vi "MainAccelerometer.vi"() -> ()   [LabVIEW 2014]
uses:
  <vilib>/myRIO/Instrument Drivers/Onboard Devices/Accelerometer/typedefs/Accelerometer Reference.ctl
  <vilib>/myRIO/Common/Instrument Driver Framework/Utilities/typedefs/myRIO Generic Hardware Reference.ctl
  <vilib>/myRIO/Common/Instrument Driver Framework/Utilities/typedefs/Hardware Version Enum.ctl
  <vilib>/myRIO/Common/Instrument Driver Framework/Utilities/typedefs/myRIO v1.0 Reference.ctl
  <vilib>/myRIO/Common/Instrument Driver Framework/Utilities/typedefs/Generic FPGA Reference.ctl
  <vilib>/myRIO/Common/Instrument Driver Framework/myRIO v1.0/Accelerometer/typedefs/Accelerometer Channels List.ctl
  <vilib>/myRIO/Common/Instrument Driver Framework/myRIO v1.0/Accelerometer/typedefs/Accelerometer Channels Enum.ctl
  <vilib>/userdefined/High Color/nirio_resource_hc.ctl
  <vilib>/myRIO/Common/Instrument Driver Framework/Utilities/vis/Is FPGA Ref Available.vi
  <vilib>/myRIO/Common/Instrument Driver Framework/myRIO v1.0/Accelerometer/vis/myRIO v1.1 Open Accelerometer.vi
  <vilib>/myRIO/Instrument Drivers/Onboard Devices/Accelerometer/vis/Read.vi
  <vilib>/myRIO/Common/Instrument Driver Framework/Utilities/vis/Validate Channels.vi
  <vilib>/myRIO/Common/Instrument Driver Framework/myRIO v1.0/Accelerometer/vis/myRIO v1.0 Reserve Accelerometer.vi
  <vilib>/myRIO/Common/Instrument Driver Framework/myRIO v1.0/UART/vis/myRIO v1.0 Close UART.vi
  <vilib>/myRIO/Common/Instrument Driver Framework/myRIO v1.0/Resource Manager/vis/myRIO v1.0 Reserve Channel List.vi
  <vilib>/myRIO/Common/Instrument Driver Framework/myRIO v1.0/Accelerometer/vis/myRIO v1.0 Build MUX Configuration Accelerometer.vi
  <vilib>/myRIO/Common/Instrument Driver Framework/myRIO v1.0/Resource Manager/vis/myRIO v1.0 Reserve Channel.vi
  <vilib>/myRIO/Common/Instrument Driver Framework/myRIO v1.0/Resource Manager/vis/myRIO v1.0 Unreserve Channel.vi
  <vilib>/myRIO/Common/Instrument Driver Framework/myRIO v1.0/Resource Manager/vis/myRIO v1.0 Build Mutex Name.vi
  <vilib>/Utility/VariantDataType/GetNumericInfo.vi
  <vilib>/Utility/error.llb/Error Cluster From Error Code.vi
  <vilib>/myRIO/Common/Instrument Driver Framework/myRIO v1.0/myRIO v1.1 Open.vi
  <vilib>/myRIO/Common/Instrument Driver Framework/myRIO v1.0/Accelerometer/vis/myRIO v1.0 Get Scaling Constant Accelerometer.vi
  <vilib>/myRIO/Common/Instrument Driver Framework/Utilities/vis/IO Manager.vi
  <vilib>/myRIO/Common/Instrument Driver Framework/Utilities/vis/Configuration Manager.vi
  <vilib>/myRIO/Common/Instrument Driver Framework/myRIO v1.0/myRIO v1.0 Close.vi
  <vilib>/myRIO/Common/Instrument Driver Framework/myRIO v1.0/Accelerometer/vis/myRIO v1.0 Read Accelerometer.vi
  <vilib>/myRIO/Common/Instrument Driver Framework/Utilities/vis/FPGA Ref Manager.vi
  <vilib>/myRIO/Common/Instrument Driver Framework/myRIO v1.0/myRIO v1.0 Reset FPGA.vi
  <vilib>/myRIO/Common/Instrument Driver Framework/myRIO v1.0/IRQ/vis/myRIO v1.0 IRQ Info FGV.vi
  <vilib>/myRIO/Common/Instrument Driver Framework/myRIO v1.0/IRQ/vis/myRIO v1.0 Timer IRQ Info FGV.vi
  <vilib>/myRIO/Common/Instrument Driver Framework/myRIO v1.0/IRQ/vis/myRIO v1.0 ISR Agent.vi
  <vilib>/myRIO/Express VI/Onboard Devices/Accelerometer/Accelerometer Express VI.xnode
  <vilib>/myRIO/Instrument Drivers/Onboard Devices/Accelerometer/vis/myRIO Accelerometer Open.xnode
  <vilib>/myRIO/Instrument Drivers/Utilities/Utilities.lvlib
  <vilib>/myRIO/Instrument Drivers/Onboard Devices/Accelerometer/Accelerometer.lvlib
panel:
  out "Acceleration":T1(graph)
  out "error out":errorcluster
  in  "Stop Button":bool
  # "Overview: The myRIO Project template acquires acceleration data from the onboard accelerometer and displays the changes of acceleration values in a waveform chart.\nInstructions:\n1. Check the myRIO target IP Address in the project and make sure the target IP Address is correct. \n2. Run the VI."
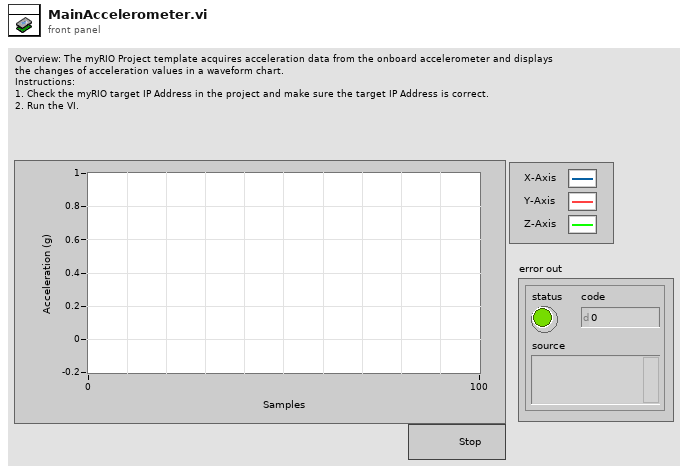
[diagram p1: front panel]
types:
  T1 = cluster{"X-Axis":dbl, "Y-Axis":dbl, "Z-Axis":dbl}
  T2 = typedef "Accelerometer.lvlib/Accelerometer Reference.ctl" = cluster{"myRIO Reference":T3, "Accelerometer Channels List":T7, "LSB Weight":dbl}
  T3 = typedef "myRIO Generic Hardware Reference.ctl" = cluster{"myRIO Model":T4, "myRIO Hardware Reference":T5}
  T4 = typedef "Hardware Version Enum.ctl" = enum16{"Unknown", "myRIO-1900", "myRIO-1950"}
  T5 = typedef "myRIO v1.0 Reference.ctl" = cluster{"Generic FPGA Reference":T6, "Allow multiple opens":bool}
  T6 = typedef "Generic FPGA Reference.ctl" = refnum<k20>
  T7 = typedef "Accelerometer Channels List.ctl" = T8[]
  T8 = typedef "Accelerometer Channels Enum.ctl" = enum16{"Not Connected", "X-Axis", "Y-Axis", "Z-Axis"}
  T9 = typedef "nirio_resource_hc.ctl" = tag
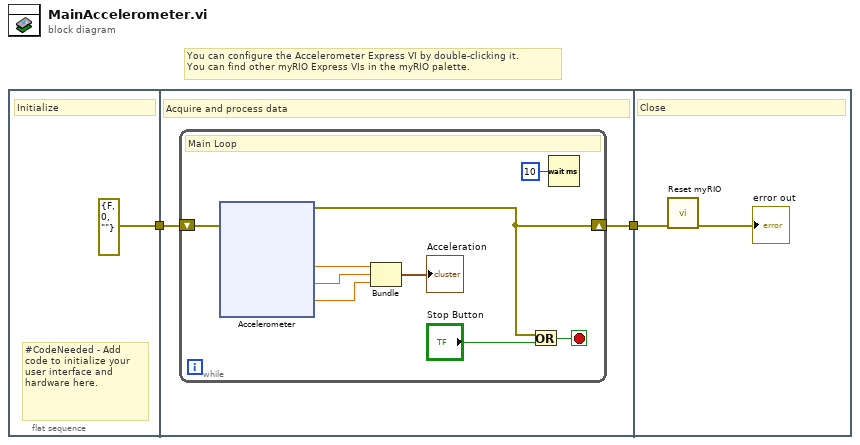
[diagram p0: block diagram]
diagram:
  # "You can configure the Accelerometer Express VI by double-clicking it.\nYou can find other myRIO Express VIs in the myRIO palette."
  n1 = flat-sequence {
    tunnel: [errorcluster {"status"=FALSE, "code"=0, "source"=""} ("error out")] -> w2
    tunnel: w2 -> [w5]
    tunnel: [w4] -> w1
    tunnel: w1 -> [w55]
    frame #0 {
      # "#CodeNeeded - Add code to initialize your user interface and hardware here."
      # "Initialize"
    }
    frame #1 {
      # "Acquire and process data"
      n2 = while {
        shift-right: [w9] -> w4
        shift-left: w5 -> [w10]
        stop <- w13 stop-if-true
        # "Main Loop"
        n3 = xnode "Accelerometer"("error in (no error)"=w10) -> ("X-Axis"=w8:dbl, "Y-Axis"=w7:dbl, "Z-Axis"=w6:dbl, "error out"=w9:errorcluster)
        n4 = Bundle("X-Axis"=w8, "Y-Axis"=w7, "Z-Axis"=w6) -> (→"Acceleration":T1)  [unwired: 1 in]
        n5 = Or(x=w9, y="Stop Button") -> (x .or. y?=w13:bool)
        n6 = Wait (ms)(milliseconds to wait=u32 10) -> ()  [unwired: 1 out]
      }
    }
    frame #2 {
      # "Close"
      n7 = call <vilib>:"Reset myRIO.vi"("error in (no error)"=w55) -> ("error out"=→"error out":errorcluster)  [unwired: 10 in]
    }
  }
